vi "TEST_ASIC_SUMnADDS_NEW.vi"(0 "Instrument VISA in":T1={"AWG VISA"="generadorpulsos", "Oscilloscope  VISA "="Oscilloscope", "Integration Board IP"="172.16.7.43", "connection ID"=refnum, "report out"=refnum, "report file path"=path "C:/Documents and Settings/CTA_LAB01/Desktop/L0_Asic/L0 Asic Test Data"}, 2 "Serial number":string="SN018", 11 "error in":errorcluster) -> (4 "Instrument VISA out":T1={"AWG VISA"="generadorpulsos", "Oscilloscope  VISA "="Oscilloscope", "Integration Board IP"="172.16.7.43", "connection ID"=refnum, "report out"=refnum, "report file path"=path "C:/Documents and Settings/CTA_LAB01/Desktop/L0_Asic/L0 Asic Test Data"}, 15 "error out":errorcluster)   [LabVIEW 2009]
uses:
  <vilib>/Utility/NIReport.llb/NI_report.lvclass
  <vilib>/Utility/NIReport.llb/HTML/NI_HTML.lvclass
  Sum_Abrilader/L0_Sum_Adder Folder/C/Program Files/National Instruments/LabVIEW 2012/instr.lib/Agilent 81150/Agilent 81150.lvlib
  <instrlib>/Agilent 8000 Series/Agilent 8000 Series.lvlib
panel:
  in  "NChannels":i32[](array[numeric])=[2, 2, 2, 2, 3, 3, 3, 4, 4, 5, 5, 6, 6, 7]
  in  "Channels Combinations":i32[](array[numeric])=[3, 12, 48, 96, 7, 28, 112, 15, 120, 31, 124, 63, 126, 127]
  out "Filename Out":path=path "C:/Documents and Settings/CTA_LAB01/Desktop/L0_Asic/L0 Asic Test Data/SN018_SumnAdds_Test.lvm"
  out "points quantity":dbl=146.0
  out "appended array":dbl[](array[numeric])=[0.2, 127.0, 63.0, 0.0, 1.0, 9.99999e+37, 9.99999e+37, 2.156e-09, 1.2e-11, 9.99999e+37, 9.99999e+37, 2.647e-09, 9e-12, 1.023e-08, 2.6e-11, 146.0]
  out "read buffer 3":string="V amptd(1),9.99999E+37,9.99999E+37,9.99999E+37,9.99999E+37,9.99999E+37,1.46E+02,+ width(1),2.14E-09,2.12E-09,2.18E-09,2.156E-09,1.2E-11,1.46E+02,V amptd(f2),9.99999E+37,9.99999E+37,9.99999E+37,9.99999E+37,9.99999E+37,1.46E+02,+ width(f2),2.64E-09,2.62E-09,2.68E-09,2.647E-09,9E-12,1.46E+02,Time(1-f2),1.022E-08,1.020E-08,1.034E-08,1.0230E-08,2.6E-11,1.46E+02\n"
  in  "Voltage":dbl[](array[numeric])=[0.05, 0.2]
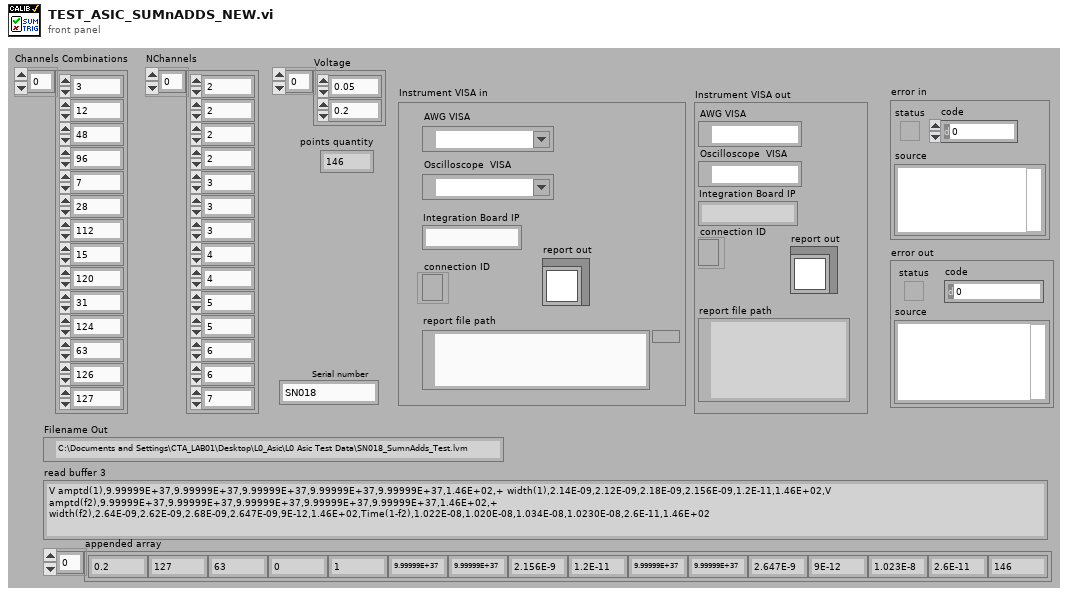
[diagram p1: front panel]
types:
  T1 = cluster{"AWG VISA":refnum<visa-resource-name>, "Oscilloscope  VISA ":refnum<visa-resource-name>, "Integration Board IP":string, "connection ID":refnum<k5>, "report out":refnum<class "NI_report.lvclass">, "report file path":path}
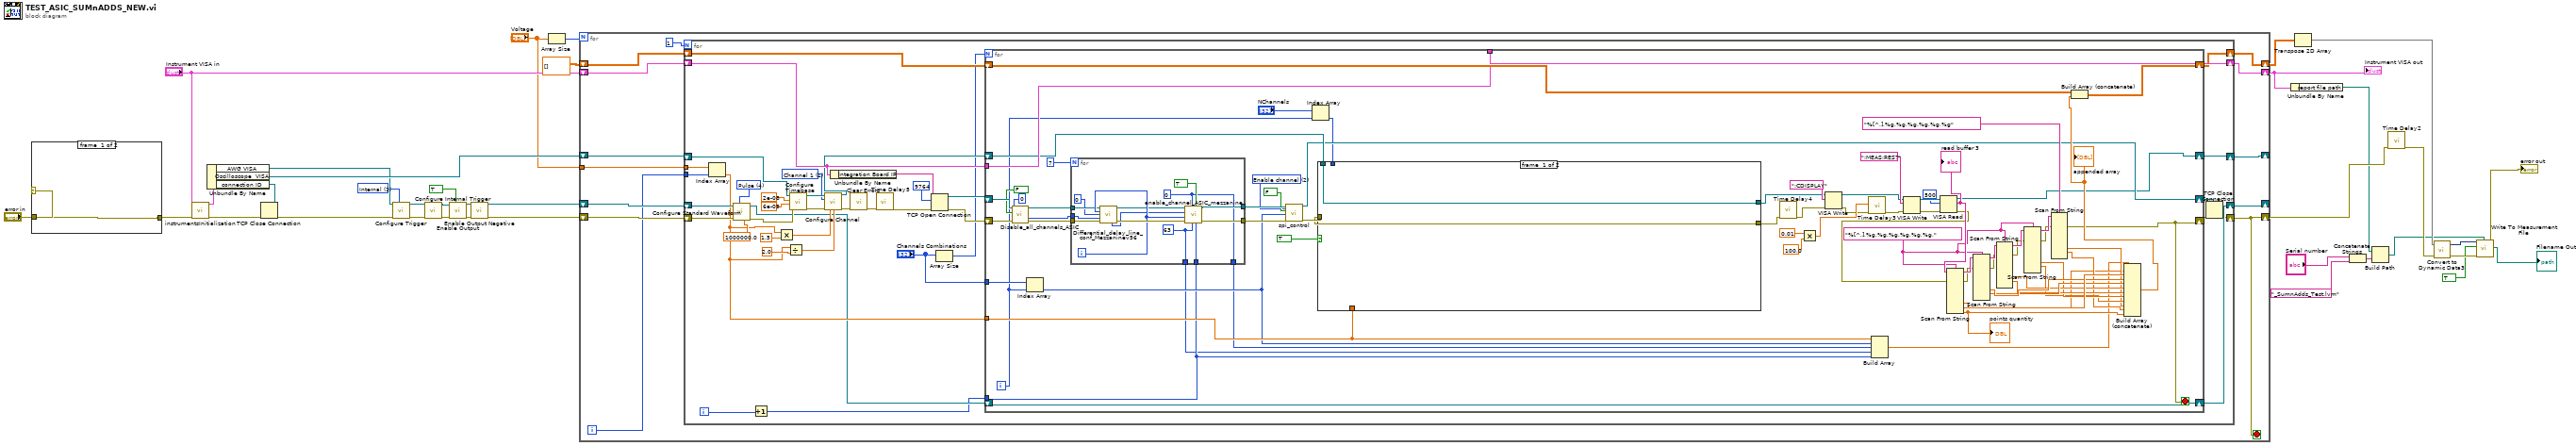
[diagram p0: block diagram]
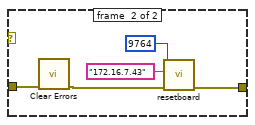
[diagram p2: hidden frame]
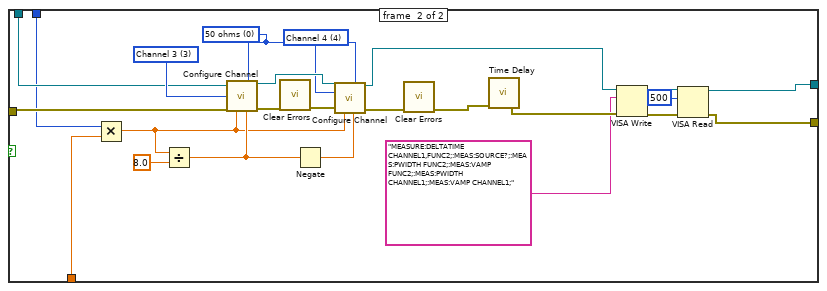
[diagram p3: hidden frame]
diagram:
  w18 = u16 1 items=["Immediate", "Internal", "External", "Software Trigger Function"] ("Trigger Source (0: Immediate)")
  n1 = case shown="Error" "error in" {
    tunnel: "error in" -> [w37 w39]
    tunnel: [w37 w42] -> w14
    frame #0 {
    }
    frame #1 {
      n2 = call <vilib>:"Clear Errors.vi"("error in (no error)"=w39) -> ("error out"=w38:errorcluster)  [unwired: 6 in]
      n3 = call "resetboard.vi"("error in (no error)"=w38, "address"="172.16.7.43", "remote port or service name"=u16 9764) -> ("error out"=w42:errorcluster)  [unwired: 7 in, 1 out]
    }
  }
  n4 = call "instrumentsInitialization.vi"("error in"=w14, "Instrument VISA in"="Instrument VISA in") -> ("error out"=w12:errorcluster, "Instrument VISA out"=w33:T1)  [unwired: 8 in]
  n5 = Unbundle By Name(w33) -> ("AWG VISA"=w21:refnum<visa-resource-name>, "Oscilloscope  VISA"=w32:refnum<visa-resource-name>, "connection ID"=w13:refnum<k5>)
  n6 = TCP Close Connection(connection ID=w13, error in (no error)=w12) -> (error out=w1:errorcluster)  [unwired: 1 in, 1 out]
  n7 = call <instrlib>:"Configure Trigger.vi"("Trigger Source (0: Immediate)"=w18, "error in (no error)"=w1, "VISA resource name"=w21) -> ("error out"=w19:errorcluster, "VISA resource name out"=w20:refnum<visa-resource-name>)  [unwired: 7 in]
  n8 = call <instrlib>:"Configure Internal Trigger.vi"("error in (no error)"=w19, "VISA resource name"=w20) -> ("error out"=w22:errorcluster, "VISA resource name out"=w23:refnum<visa-resource-name>)  [unwired: 8 in]
  n9 = call <instrlib>:"Enable Output.vi"("Enable Output (T: Enable)"=TRUE, "error in (no error)"=w22, "VISA resource name"=w23) -> ("error out"=w10:errorcluster, "VISA resource name out"=w9:refnum<visa-resource-name>)  [unwired: 7 in]
  n10 = call <instrlib>:"Enable Output Negative.vi"("error in (no error)"=w10, "VISA resource name"=w9) -> ("error out"=w2:errorcluster, "VISA resource name out"=w11:refnum<visa-resource-name>)  [unwired: 8 in]
  n11 = Array Size(array="Voltage") -> (size(s)=w34:i32)
  n12 = for {
    N: w34 -> [_]
    shift-right: [w43] -> w25
    shift-left: w2 -> [w55]
    tunnel: "Voltage" -> [w53]
    shift-right: [w48] -> w24
    shift-left: "Instrument VISA in" -> [w50]
    shift-right: [w47] -> w28
    shift-left: dbl[][] [] -> [w49]
    shift-right: [w44] -> _
    shift-left: w11 -> [w54]
    shift-right: [w45] -> _
    shift-left: w32 -> [w51]
    i -> [w52]
    stop <- w43 stop-if-true
    n13 = for {
      N: 1 -> [_]
      tunnel: w53 -> [w91]
      tunnel: w52 -> [w90]
      shift-right: [w66] -> w47
      shift-left: w49 -> [w69]
      shift-right: [w67] -> w48
      shift-left: w50 -> [w79]
      shift-right: [w62] -> w43
      shift-left: w55 -> [w93]
      shift-right: [w63] -> w44
      shift-left: w54 -> [w92]
      shift-right: [w65] -> w45
      shift-left: w51 -> [w86]
      i -> [w57]
      w82 = 1 items=["Channel 1"=1, "Channel 2"=2, "Channel 3"=3, "Channel 4"=4] ("Channel (1: Channel 1)")
      w95 = u16 4 items=["Sine", "Square", "Ramp Up", "Ramp Down", "Pulse", "Noise", "DC"] ("Waveform (0: Sine)")
      n14 = Index Array(array=w91, index=w90) -> (element=w68:dbl)
      n15 = call <instrlib>:"Configure Standard Waveform.vi"("Frequency (1000.0 Hz)"=1000000.0, "Waveform (0: Sine)"=w95, "error in (no error)"=w93, "Amplitude (1.0 Vpp)"=w68, "VISA resource name"=w92) -> ("error out"=w89:errorcluster, "VISA resource name out"=w64:refnum<visa-resource-name>)  [unwired: 5 in]
      n16 = Increment(x=w57) -> (x+1=w56:i32)
      n17 = Multiply(x=w68, y=1.5) -> (x*y=w81:dbl)
      n18 = Divide(x=w68, y=2.0) -> (x/y=w74:dbl)
      n19 = call <instrlib>:"Configure Timebase.vi"("error in (no error)"=w89, "Position (0.0 s)"=6e-09, "Timebase (0.005 s)"=2e-08, "VISA resource name"=w86) -> ("error out"=w88:errorcluster, "VISA resource name out"=w85:refnum<visa-resource-name>)  [unwired: 6 in]
      n20 = call <instrlib>:"Configure Channel.vi"("VISA resource name"=w85, "Channel (1: Channel 1)"=w82, "error in (no error)"=w88, "Vertical Range (2.0 V)"=w81, "Vertical Offset (0.0 V)"=w74) -> ("VISA resource name out"=w73:refnum<visa-resource-name>, "error out"=w87:errorcluster)  [unwired: 9 in]
      n21 = Unbundle By Name(w79) -> ("Integration Board IP"=w77:string)
      n22 = call <vilib>:"Clear Errors.vi"("error in (no error)"=w87) -> ("error out"=w61:errorcluster)  [unwired: 6 in]
      n23 = call "Time Delay5"("error in (no error)"=w61) -> ("error out"=w60:errorcluster)  [unwired: 10 in]
      n24 = TCP Open Connection(address=w77, remote port or service name=u16 9764, error in (no error)=w60) -> (connection ID=w70:refnum<k5>, error out=w78:errorcluster)  [unwired: 2 in]
      n25 = Array Size(array="Channels Combinations") -> (size(s)=w59:i32)
      n26 = for {
        N: w59 -> [_]
        shift-right: [w122] -> w72
        shift-left: w78 -> [w162]
        tunnel: w79 -> [w161]
        tunnel: [w161] -> w67
        shift-right: [w163] -> w66
        shift-left: w69 -> [w164]
        shift-right: [w123] -> w71
        shift-left: w70 -> [w121]
        tunnel: w68 -> [w113]
        tunnel: w56 -> [w106]
        shift-right: [w118] -> w65
        shift-left: w73 -> [w159]
        shift-right: [w117] -> w63
        shift-left: w64 -> [w117]
        tunnel: "Channels Combinations" -> [w109]
        i -> [w102]
        stop <- w122 stop-if-true
        w104 = u16 2 items=["Attenuation", "Clipping", "Enable channel", "Delay line", "ASIC"] ("Device")
        w144 = "%[^,],%g,%g,%g,%g,%g,%g," ("format string")
        n27 = call "Disable_all_channels_ASIC.vi"("error in"=w162, "id_in"=0 ("Data"), "Clip_en_b"=FALSE, "connection ID"=w121) -> ("error out"=w97:errorcluster, "id_out"=w96:i32, "connection ID out"=w98:refnum<k5>)  [unwired: 5 in]
        n28 = Index Array(array=w109, index=w102) -> (element=w108:i32)
        n29 = for {
          N: 7 -> [_]
          tunnel: w97 -> [w173]
          tunnel: w98 -> [w170]
          tunnel: [w178] -> w112
          tunnel: [w177] -> w111
          tunnel: [w176] -> w100
          tunnel: [w175] -> w99
          tunnel: w106 -> [w174]
          tunnel: w96 -> [w167]
          i -> [w171]
          w176 = u32 0 ("Att gain")
          w175 = u32 63 ("Ib_clipVb")
          n30 = call "Differential_delay_line_conf_Mezzaninev56.vi"("connection ID"=w170, "channel"=w171, "Delay value"=u16 0, "Id in"=w167, "error in (no error)"=w173) -> ("connection ID out"=w169:refnum<k5>, "Id out"=w166:i32, "error out 2"=w172:errorcluster)  [unwired: 3 in, 5 out]
          n31 = call "enable_channel_ASIC_mezzanine.vi"("Clip_sel_b"=w174, "maj/sum"=TRUE, "Ib_clipVb"=w175, "Att gain"=w176, "error in"=w172, "Channel"=w171, "id_in"=w166, "connection ID"=w169) -> ("error out"=w177:errorcluster, "connection ID out"=w178:refnum<k5>)  [unwired: 1 in, 1 out]
        }
        n32 = call "spi_control.vi"("connection ID"=w112, "Device"=w104, "Read/#write"=FALSE, "Data"=w108, "error out 3"=w111) -> ("connection ID out"=w123:refnum<k5>, "error out 2"=w160:errorcluster)  [unwired: 7 in, 6 out]
        n33 = Index Array(array="NChannels", index=w102) -> (element=w101:i32)
        n34 = case shown="True" TRUE ("maj/sum") {
          tunnel: [w181 w192] -> w114
          tunnel: w160 -> [w181 w187]
          tunnel: w159 -> [w180 w188]
          tunnel: [w180 w198] -> w126
          tunnel: w113 -> [_ w184]
          tunnel: w101 -> [_ w183]
          frame #0 {
          }
          frame #1 {
            w199 = u32 0 items=["50 ohms", "1 Mohms"] ("Input Impedance (1: 1 Mohms)")
            w191 = 3 items=["Channel 1"=1, "Channel 2"=2, "Channel 3"=3, "Channel 4"=4] ("Channel (1: Channel 1)")
            w190 = 4 items=["Channel 1"=1, "Channel 2"=2, "Channel 3"=3, "Channel 4"=4] ("Channel (1: Channel 1)")
            n35 = Multiply(x=w183, y=w184) -> (x*y=w182:dbl)
            n36 = Divide(x=w182, y=8.0) -> (x/y=w185:dbl)
            n37 = call <instrlib>:"Configure Channel.vi"("VISA resource name"=w188, "Input Impedance (1: 1 Mohms)"=w199, "Channel (1: Channel 1)"=w191, "error in (no error)"=w187, "Vertical Range (2.0 V)"=w182, "Vertical Offset (0.0 V)"=w185) -> ("VISA resource name out"=w203:refnum<visa-resource-name>, "error out"=w205:errorcluster)  [unwired: 8 in]
            n38 = call <vilib>:"Clear Errors.vi"("error in (no error)"=w205) -> ("error out"=w197:errorcluster)  [unwired: 6 in]
            n39 = Negate(x=w185) -> (-x=w189:dbl)
            n40 = call <instrlib>:"Configure Channel.vi"("VISA resource name"=w203, "Input Impedance (1: 1 Mohms)"=w199, "Channel (1: Channel 1)"=w190, "error in (no error)"=w197, "Vertical Range (2.0 V)"=w182, "Vertical Offset (0.0 V)"=w189) -> ("VISA resource name out"=w195:refnum<visa-resource-name>, "error out"=w204:errorcluster)  [unwired: 8 in]
            n41 = call <vilib>:"Clear Errors.vi"("error in (no error)"=w204) -> ("error out"=w196:errorcluster)  [unwired: 6 in]
            n42 = call "Time Delay"("error in (no error)"=w196) -> ("error out"=w194:errorcluster)  [unwired: 10 in]
            n43 = VISA Write(VISA resource name=w195, write buffer="MEASURE:DELTATIME CHANNEL1,FUNC2;:MEAS:SOURCE?;:MEAS:PWIDTH FUNC2;:MEAS:VAMP FUNC2;:MEAS:PWIDTH CHANNEL1;:MEAS:VAMP CHANNEL1;", error in (no error)=w194) -> (VISA resource name out=w202:refnum<visa-resource-name>, error out=w201:errorcluster)  [unwired: 1 out]
            n44 = VISA Read(VISA resource name=w202, byte count=u32 500, error in (no error)=w201) -> (VISA resource name out=w198:refnum<visa-resource-name>, error out=w192:errorcluster)  [unwired: 2 out]
          }
        }
        n45 = call "Time Delay4"("error in (no error)"=w114) -> ("error out"=w115:errorcluster)  [unwired: 10 in]
        n46 = Multiply(x=0.01, y=100.0) -> (x*y=w151:dbl)
        n47 = VISA Write(VISA resource name=w126, write buffer=":CDISPLAY", error in (no error)=w115) -> (VISA resource name out=w129:refnum<visa-resource-name>, error out=w127:errorcluster)  [unwired: 1 out]
        n48 = call "Time Delay3"("error in (no error)"=w127, "Delay Time (s)"=w151) -> ("error out"=w150:errorcluster)  [unwired: 9 in]
        n49 = Build Array(w113, w108, w100, w99, w106) -> (w119:dbl[])
        n50 = VISA Write(VISA resource name=w129, write buffer=":MEAS:RES?", error in (no error)=w150) -> (VISA resource name out=w158:refnum<visa-resource-name>, error out=w157:errorcluster)  [unwired: 1 out]
        n51 = VISA Read(VISA resource name=w158, byte count=u32 500, error in (no error)=w157) -> (VISA resource name out=w118:refnum<visa-resource-name>, read buffer=w154:string, error out=w134:errorcluster)  [unwired: 1 out]
        "read buffer 3" <- w154
        n52 = Scan From String(format string=w144, input string=w154, error in=w134) -> (remaining string=w148:string, error out=w130:errorcluster, output 5=w120:dbl, output 6=w149:dbl, output 7=w135:dbl)  [unwired: 12 in, 1 out]
        "points quantity" <- w135
        n53 = Scan From String(format string=w144, input string=w148, error in=w130) -> (remaining string=w145:string, error out=w131:errorcluster, output 5=w142:dbl, output 6=w141:dbl)  [unwired: 13 in, 1 out]
        n54 = Scan From String(format string=w144, input string=w145, error in=w131) -> (remaining string=w146:string, error out=w132:errorcluster, output 5=w140:dbl, output 6=w139:dbl)  [unwired: 13 in, 1 out]
        n55 = Scan From String(format string=w144, input string=w146, error in=w132) -> (remaining string=w147:string, error out=w133:errorcluster, output 5=w138:dbl, output 6=w137:dbl)  [unwired: 13 in, 1 out]
        n56 = Scan From String(format string="%[^,],%g,%g,%g,%g,%g,%g", input string=w147, error in=w133) -> (error out=w122:errorcluster, output 5=w125:dbl, output 6=w136:dbl)  [unwired: 13 in, 2 out]
        n57 = Build Array (concatenate)(w119, w120, w149, w142, w141, w140, w139, w138, w137, w125, w136, w135) -> (w124:dbl[])
        "appended array" <- w124
        n58 = Build Array (concatenate)(w164, w124) -> (w163:dbl[][])
      }
      n59 = TCP Close Connection(connection ID=w71, error in (no error)=w72) -> (error out=w62:errorcluster)  [unwired: 1 in, 1 out]
    }
  }
  "Instrument VISA out" <- w24
  n60 = Unbundle By Name(w24) -> ("report file path"=w4:path)
  n61 = Transpose 2D Array(2D array=w28) -> (transposed array=w16:dbl[][])
  n62 = Concatenate Strings("Serial number", "_SumnAdds_Test.lvm" ("name or relative path")) -> (w30:string)
  n63 = Build Path(base path=w4, name or relative path=w30) -> (appended path=w3:path)
  n64 = call "Time Delay2"("error in (no error)"=w25) -> ("error out"=w35:errorcluster)  [unwired: 10 in]
  n65 = call "Convert to Dynamic Data3"("2D Array"=w16) -> ("Dynamic Data Type"=w17:dynamicdata)  [unwired: 3 in]
  n66 = call "Write To Measurement File"("Signals"=w17, "Enable"=TRUE, "error in (no error)"=w35, "Filename"=w3) -> ("Filename Out"=→"Filename Out":path, "error out"=→"error out":errorcluster)  [unwired: 13 in, 1 out]
